vi "Motion configurations.vi"(9 "Motion config now":string="rLscaleL.xml") -> (2 "Array":T1[](array[typedef])=[{"Distance (ft)"=24.4, "Angle (degrees)"=0.0, "Time (s)"=0.5, "Intake Mode"=enum."Nothing", "Shooting Mode"=enum."No Shooter"}, {"Distance (ft)"=0.0, "Angle (degrees)"=45.0, "Time (s)"=0.5, "Intake Mode"=enum."Nothing", "Shooting Mode"=enum."No Shooter"}, {"Distance (ft)"=1.0, "Angle (degrees)"=0.0, "Time (s)"=0.0, "Intake Mode"=enum."Nothing", "Shooting Mode"=enum."No Shooter"}, {"Distance (ft)"=0.0, "Angle (degrees)"=45.0, "Time (s)"=0.0, "Intake Mode"=enum."Nothing", "Shooting Mode"=enum."No Shooter"}, {"Distance (ft)"=0.0, "Angle (degrees)"=0.0, "Time (s)"=0.0, "Intake Mode"=enum."Nothing", "Shooting Mode"=enum."High Scale Shooter"}])   [LabVIEW 2017]
uses:
  Auton Control.ctl
panel:
  in  "Motion configs":cluster{"Motion config":string, "Array":T1[]}[](array[cluster])=[{"Motion config"="Straight.xml", "Array"=[{"Distance (ft)"=7.5, "Angle (degrees)"=0.0, "Time (s)"=0.0, "Intake Mode"=enum."Nothing", "Shooting Mode"=enum."No Shooter"}]}, {"Motion config"="rCscaleL.xml", "Array"=[{"Distance (ft)"=3.5, "Angle (degrees)"=0.0, "Time (s)"=0.5, "Intake Mode"=enum."Nothing", "Shooting Mode"=enum."No Shooter"}, {"Distance (ft)"=0.0, "Angle (degrees)"=-90.0, "Time (s)"=0.5, "Intake Mode"=enum."Nothing", "Shooting Mode"=enum."No Shooter"}, {"Distance (ft)"=10.0, "Angle (degrees)"=0.0, "Time (s)"=0.5, "Intake Mode"=enum."Nothing", "Shooting Mode"=enum."No Shooter"}, {"Distance (ft)"=0.0, "Angle (degrees)"=90.0, "Time (s)"=0.5, "Intake Mode"=enum."Nothing", "Shooting Mode"=enum."No Shooter"}, {"Distance (ft)"=20.9, "Angle (degrees)"=0.0, "Time (s)"=0.5, "Intake Mode"=enum."Nothing", "Shooting Mode"=enum."No Shooter"}, {"Distance (ft)"=0.0, "Angle (degrees)"=90.0, "Time (s)"=0.5, "Intake Mode"=enum."Nothing", "Shooting Mode"=enum."No Shooter"}, {"Distance (ft)"=0.0, "Angle (degrees)"=0.0, "Time (s)"=0.0, "Intake Mode"=enum."Nothing", "Shooting Mode"=enum."Mid Scale Shooter"}]}, {"Motion config"="rCscaleR.xml", "Array"=[{"Distance (ft)"=3.5, "Angle (degrees)"=0.0, "Time (s)"=0.5, "Intake Mode"=enum."Nothing", "Shooting Mode"=enum."No Shooter"}, {"Distance (ft)"=0.0, "Angle (degrees)"=90.0, "Time (s)"=0.5, "Intake Mode"=enum."Nothing", "Shooting Mode"=enum."No Shooter"}, {"Distance (ft)"=7.0, "Angle (degrees)"=0.0, "Time (s)"=0.5, "Intake Mode"=enum."Nothing", "Shooting Mode"=enum."No Shooter"}, {"Distance (ft)"=0.0, "Angle (degrees)"=-90.0, "Time (s)"=0.5, "Intake Mode"=enum."Nothing", "Shooting Mode"=enum."No Shooter"}, {"Distance (ft)"=20.9, "Angle (degrees)"=0.0, "Time (s)"=0.5, "Intake Mode"=enum."Nothing", "Shooting Mode"=enum."No Shooter"}, {"Distance (ft)"=0.0, "Angle (degrees)"=-90.0, "Time (s)"=0.5, "Intake Mode"=enum."Nothing", "Shooting Mode"=enum."No Shooter"}, {"Distance (ft)"=0.0, "Angle (degrees)"=0.0, "Time (s)"=0.0, "Intake Mode"=enum."Nothing", "Shooting Mode"=enum."Mid Scale Shooter"}]}, {"Motion config"="rCswitchL.xml", "Array"=[{"Distance (ft)"=1.5, "Angle (degrees)"=0.0, "Time (s)"=0.5, "Intake Mode"=enum."Nothing", "Shooting Mode"=enum."No Shooter"}, {"Distance (ft)"=0.0, "Angle (degrees)"=-45.0, "Time (s)"=0.5, "Intake Mode"=enum."Nothing", "Shooting Mode"=enum."No Shooter"}, {"Distance (ft)"=6.0, "Angle (degrees)"=0.0, "Time (s)"=0.5, "Intake Mode"=enum."Nothing", "Shooting Mode"=enum."No Shooter"}, {"Distance (ft)"=0.0, "Angle (degrees)"=45.0, "Time (s)"=0.5, "Intake Mode"=enum."Nothing", "Shooting Mode"=enum."No Shooter"}, {"Distance (ft)"=3.0, "Angle (degrees)"=0.0, "Time (s)"=0.5, "Intake Mode"=enum."Nothing", "Shooting Mode"=enum."No Shooter"}, {"Distance (ft)"=0.5, "Angle (degrees)"=0.0, "Time (s)"=0.0, "Intake Mode"=enum."Nothing", "Shooting Mode"=enum."Switch Shooter"}]}, {"Motion config"="rCswitchR.xml", "Array"=[{"Distance (ft)"=1.5, "Angle (degrees)"=0.0, "Time (s)"=0.5, "Intake Mode"=enum."Nothing", "Shooting Mode"=enum."No Shooter"}, {"Distance (ft)"=0.0, "Angle (degrees)"=45.0, "Time (s)"=0.5, "Intake Mode"=enum."Nothing", "Shooting Mode"=enum."No Shooter"}, {"Distance (ft)"=5.5, "Angle (degrees)"=0.0, "Time (s)"=0.5, "Intake Mode"=enum."Nothing", "Shooting Mode"=enum."No Shooter"}, {"Distance (ft)"=0.0, "Angle (degrees)"=-45.0, "Time (s)"=0.5, "Intake Mode"=enum."Nothing", "Shooting Mode"=enum."No Shooter"}, {"Distance (ft)"=3.0, "Angle (degrees)"=0.0, "Time (s)"=0.5, "Intake Mode"=enum."Nothing", "Shooting Mode"=enum."No Shooter"}, {"Distance (ft)"=0.5, "Angle (degrees)"=0.0, "Time (s)"=0.0, "Intake Mode"=enum."Nothing", "Shooting Mode"=enum."Switch Shooter"}]}, {"Motion config"="rLscaleL.xml", "Array"=[{"Distance (ft)"=24.4, "Angle (degrees)"=0.0, "Time (s)"=0.5, "Intake Mode"=enum."Nothing", "Shooting Mode"=enum."Reverse"}, {"Distance (ft)"=0.0, "Angle (degrees)"=45.0, "Time (s)"=0.5, "Intake Mode"=enum."Nothing", "Shooting Mode"=enum."No Shooter"}, {"Distance (ft)"=1.0, "Angle (degrees)"=0.0, "Time (s)"=0.0, "Intake Mode"=enum."Nothing", "Shooting Mode"=enum."No Shooter"}, {"Distance (ft)"=0.0, "Angle (degrees)"=45.0, "Time (s)"=0.0, "Intake Mode"=enum."Nothing", "Shooting Mode"=enum."No Shooter"}, {"Distance (ft)"=0.0, "Angle (degrees)"=0.0, "Time (s)"=0.0, "Intake Mode"=enum."Nothing", "Shooting Mode"=enum."High Scale Shooter"}]}, {"Motion config"="rLscaleR.xml", "Array"=[{"Distance (ft)"=3.5, "Angle (degrees)"=0.0, "Time (s)"=0.5, "Intake Mode"=enum."Nothing", "Shooting Mode"=enum."No Shooter"}, {"Distance (ft)"=0.0, "Angle (degrees)"=90.0, "Time (s)"=0.5, "Intake Mode"=enum."Nothing", "Shooting Mode"=enum."No Shooter"}, {"Distance (ft)"=17.0, "Angle (degrees)"=0.0, "Time (s)"=0.5, "Intake Mode"=enum."Nothing", "Shooting Mode"=enum."No Shooter"}, {"Distance (ft)"=0.0, "Angle (degrees)"=-90.0, "Time (s)"=0.5, "Intake Mode"=enum."Nothing", "Shooting Mode"=enum."No Shooter"}, {"Distance (ft)"=20.9, "Angle (degrees)"=0.0, "Time (s)"=0.5, "Intake Mode"=enum."Nothing", "Shooting Mode"=enum."No Shooter"}, {"Distance (ft)"=0.0, "Angle (degrees)"=-90.0, "Time (s)"=0.5, "Intake Mode"=enum."Nothing", "Shooting Mode"=enum."No Shooter"}, {"Distance (ft)"=0.0, "Angle (degrees)"=0.0, "Time (s)"=0.0, "Intake Mode"=enum."Nothing", "Shooting Mode"=enum."Mid Scale Shooter"}]}, {"Motion config"="rLswitchL.xml", "Array"=[{"Distance (ft)"=11.4, "Angle (degrees)"=0.0, "Time (s)"=0.5, "Intake Mode"=enum."Nothing", "Shooting Mode"=enum."No Shooter"}, {"Distance (ft)"=0.0, "Angle (degrees)"=90.0, "Time (s)"=0.5, "Intake Mode"=enum."Nothing", "Shooting Mode"=enum."No Shooter"}, {"Distance (ft)"=3.0, "Angle (degrees)"=0.0, "Time (s)"=0.5, "Intake Mode"=enum."Nothing", "Shooting Mode"=enum."No Shooter"}, {"Distance (ft)"=0.0, "Angle (degrees)"=0.0, "Time (s)"=0.0, "Intake Mode"=enum."Nothing", "Shooting Mode"=enum."Switch Shooter"}]}, {"Motion config"="rLswitchLscaleL.xml", "Array"=[{"Distance (ft)"=0.0, "Angle (degrees)"=0.0, "Time (s)"=0.0, "Intake Mode"=enum."Nothing", "Shooting Mode"=enum."No Shooter"}]}, {"Motion config"="rLswitchR.xml", "Array"=[{"Distance (ft)"=3.5, "Angle (degrees)"=0.0, "Time (s)"=0.5, "Intake Mode"=enum."Nothing", "Shooting Mode"=enum."No Shooter"}, {"Distance (ft)"=0.0, "Angle (degrees)"=90.0, "Time (s)"=0.5, "Intake Mode"=enum."Nothing", "Shooting Mode"=enum."No Shooter"}, {"Distance (ft)"=17.0, "Angle (degrees)"=0.0, "Time (s)"=0.5, "Intake Mode"=enum."Nothing", "Shooting Mode"=enum."No Shooter"}, {"Distance (ft)"=0.0, "Angle (degrees)"=-90.0, "Time (s)"=0.5, "Intake Mode"=enum."Nothing", "Shooting Mode"=enum."No Shooter"}, {"Distance (ft)"=7.9, "Angle (degrees)"=0.0, "Time (s)"=0.5, "Intake Mode"=enum."Nothing", "Shooting Mode"=enum."No Shooter"}, {"Distance (ft)"=0.0, "Angle (degrees)"=-90.0, "Time (s)"=0.5, "Intake Mode"=enum."Nothing", "Shooting Mode"=enum."No Shooter"}, {"Distance (ft)"=3.0, "Angle (degrees)"=0.0, "Time (s)"=0.5, "Intake Mode"=enum."Nothing", "Shooting Mode"=enum."No Shooter"}, {"Distance (ft)"=0.0, "Angle (degrees)"=0.0, "Time (s)"=0.0, "Intake Mode"=enum."Nothing", "Shooting Mode"=enum."Switch Shooter"}]}, {"Motion config"="rRscaleL.xml", "Array"=[{"Distance (ft)"=3.5, "Angle (degrees)"=0.0, "Time (s)"=0.5, "Intake Mode"=enum."Nothing", "Shooting Mode"=enum."No Shooter"}, {"Distance (ft)"=0.0, "Angle (degrees)"=-90.0, "Time (s)"=0.5, "Intake Mode"=enum."Nothing", "Shooting Mode"=enum."No Shooter"}, {"Distance (ft)"=17.0, "Angle (degrees)"=0.0, "Time (s)"=0.5, "Intake Mode"=enum."Nothing", "Shooting Mode"=enum."No Shooter"}, {"Distance (ft)"=0.0, "Angle (degrees)"=90.0, "Time (s)"=0.5, "Intake Mode"=enum."Nothing", "Shooting Mode"=enum."No Shooter"}, {"Distance (ft)"=20.9, "Angle (degrees)"=0.0, "Time (s)"=0.5, "Intake Mode"=enum."Nothing", "Shooting Mode"=enum."No Shooter"}, {"Distance (ft)"=0.0, "Angle (degrees)"=90.0, "Time (s)"=0.5, "Intake Mode"=enum."Nothing", "Shooting Mode"=enum."No Shooter"}, {"Distance (ft)"=0.0, "Angle (degrees)"=0.0, "Time (s)"=0.0, "Intake Mode"=enum."Nothing", "Shooting Mode"=enum."Mid Scale Shooter"}]}, {"Motion config"="rRscaleR.xml", "Array"=[{"Distance (ft)"=24.4, "Angle (degrees)"=0.0, "Time (s)"=0.5, "Intake Mode"=enum."Nothing", "Shooting Mode"=enum."Reverse"}, {"Distance (ft)"=0.0, "Angle (degrees)"=-45.0, "Time (s)"=0.5, "Intake Mode"=enum."Nothing", "Shooting Mode"=enum."No Shooter"}, {"Distance (ft)"=1.0, "Angle (degrees)"=0.0, "Time (s)"=0.5, "Intake Mode"=enum."Nothing", "Shooting Mode"=enum."No Shooter"}, {"Distance (ft)"=0.0, "Angle (degrees)"=-45.0, "Time (s)"=0.5, "Intake Mode"=enum."Nothing", "Shooting Mode"=enum."No Shooter"}, {"Distance (ft)"=0.0, "Angle (degrees)"=0.0, "Time (s)"=0.0, "Intake Mode"=enum."Nothing", "Shooting Mode"=enum."High Scale Shooter"}]}, {"Motion config"="rRswitchL.xml", "Array"=[{"Distance (ft)"=3.5, "Angle (degrees)"=0.0, "Time (s)"=0.5, "Intake Mode"=enum."Nothing", "Shooting Mode"=enum."No Shooter"}, {"Distance (ft)"=0.0, "Angle (degrees)"=-90.0, "Time (s)"=0.5, "Intake Mode"=enum."Nothing", "Shooting Mode"=enum."No Shooter"}, {"Distance (ft)"=17.0, "Angle (degrees)"=0.0, "Time (s)"=0.5, "Intake Mode"=enum."Nothing", "Shooting Mode"=enum."No Shooter"}, {"Distance (ft)"=0.0, "Angle (degrees)"=90.0, "Time (s)"=0.5, "Intake Mode"=enum."Nothing", "Shooting Mode"=enum."No Shooter"}, {"Distance (ft)"=7.9, "Angle (degrees)"=0.0, "Time (s)"=0.5, "Intake Mode"=enum."Nothing", "Shooting Mode"=enum."No Shooter"}, {"Distance (ft)"=0.0, "Angle (degrees)"=90.0, "Time (s)"=0.5, "Intake Mode"=enum."Nothing", "Shooting Mode"=enum."No Shooter"}, {"Distance (ft)"=0.0, "Angle (degrees)"=0.0, "Time (s)"=0.0, "Intake Mode"=enum."Nothing", "Shooting Mode"=enum."Switch Shooter"}]}, {"Motion config"="rRswitchR.xml", "Array"=[{"Distance (ft)"=11.4, "Angle (degrees)"=0.0, "Time (s)"=0.5, "Intake Mode"=enum."Nothing", "Shooting Mode"=enum."No Shooter"}, {"Distance (ft)"=0.0, "Angle (degrees)"=-90.0, "Time (s)"=0.5, "Intake Mode"=enum."Nothing", "Shooting Mode"=enum."No Shooter"}, {"Distance (ft)"=3.0, "Angle (degrees)"=0.0, "Time (s)"=0.5, "Intake Mode"=enum."Nothing", "Shooting Mode"=enum."No Shooter"}, {"Distance (ft)"=0.0, "Angle (degrees)"=0.0, "Time (s)"=0.0, "Intake Mode"=enum."Nothing", "Shooting Mode"=enum."Switch Shooter"}]}, {"Motion config"="Null.xml", "Array"=[{"Distance (ft)"=0.0, "Angle (degrees)"=0.0, "Time (s)"=0.0, "Intake Mode"=enum."Nothing", "Shooting Mode"=enum."No Shooter"}]}]
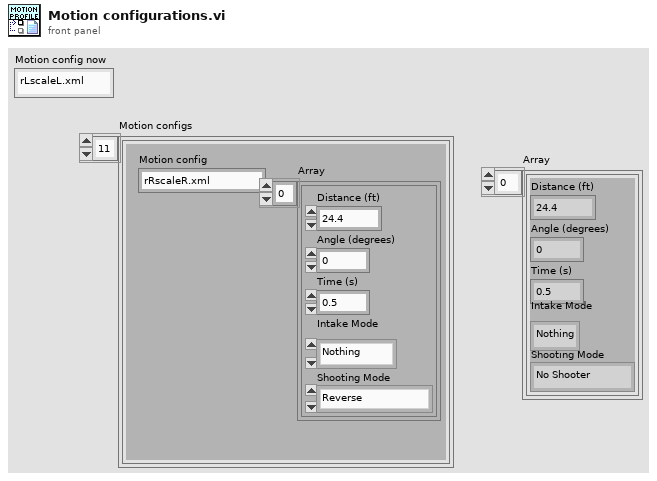
[diagram p1: front panel]
types:
  T1 = typedef "Auton Control.ctl" = cluster{"Distance (ft)":dbl, "Angle (degrees)":dbl, "Time (s)":dbl, "Intake Mode":enum16{"Nothing", "In", "Out"}, "Shooting Mode":enum16{"No Shooter", "Switch Shooter", "Low Scale Shooter", "Mid Scale Shooter", "High Scale Shooter", "Reverse"}}
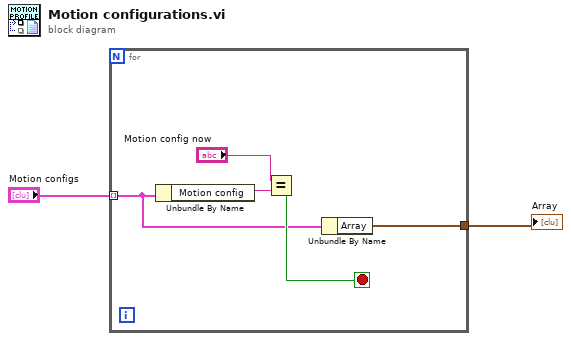
[diagram p0: block diagram]
diagram:
  n1 = for {
    tunnel: "Motion configs" -> [w4] mode=indexing
    tunnel: [w3] -> w1
    stop <- w6 stop-if-true
    n2 = Unbundle By Name(w4) -> ("Motion config"=w5:string)
    n3 = Equal?(x="Motion config now", y=w5) -> (x = y?=w6:bool)
    n4 = Unbundle By Name(w4) -> ("Array"=w3:T1[])
  }
  "Array" <- w1
